vi "vdP_measurement.vi"() -> ()   [LabVIEW 2026]
uses:
  <vilib>/regexp/Match Regular Expression.xnode
panel:
  out "rho (Ohm * m)":dbl
  out "Rs (Ohm/sq)":dbl
  in  "VISA resource name":refnum<visa-resource-name>="TCPIP0::192.168.0.4::1225::SOCKET"
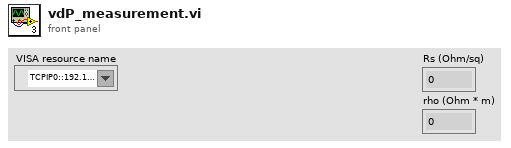
[diagram p1: front panel]
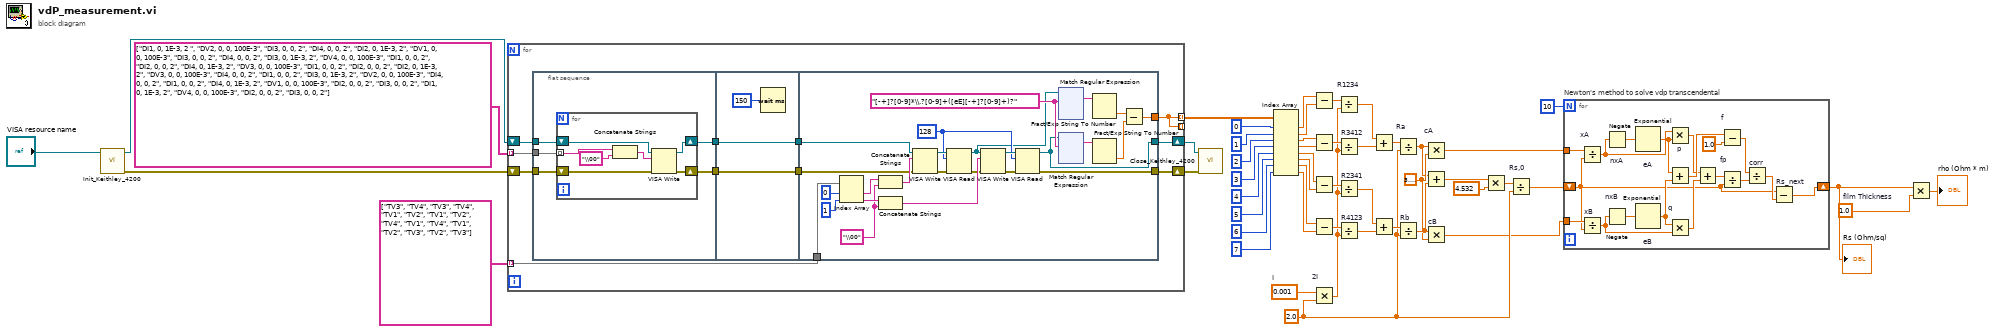
[diagram p0: block diagram]
diagram:
  w9 = 3.141592653589793
  w2 = 1.0  # film Thickness
  w34 = 0.001  # I
  w11 = 2.0 ("y")
  n1 = call "Init_Keithley_4200.vi"("VISA resource name"="VISA resource name") -> ("error out"=w46:errorcluster, "VISA resource name out"=w47:refnum<visa-resource-name>)  [unwired: 9 in]
  n2 = for {
    tunnel: string[][] [["DI1, 0, 1E-3, 2 ", "DV2, 0, 0, 100E-3", "DI3, 0, 0, 2", "DI4, 0, 0, 2"], ["DI2, 0, 1E-3, 2", "DV1, 0, 0, 100E-3", "DI3, 0, 0, 2", "DI4, 0, 0, 2"], ["DI3, 0, 1E-3, 2", "DV4, 0, 0, 100E-3", "DI1, 0, 0, 2", "DI2, 0, 0, 2"], ["DI4, 0, 1E-3, 2", "DV3, 0, 0, 100E-3", "DI1, 0, 0, 2", "DI2, 0, 0, 2"], ["DI2, 0, 1E-3, 2", "DV3, 0, 0, 100E-3", "DI4, 0, 0, 2", "DI1, 0, 0, 2"], ["DI3, 0, 1E-3, 2", "DV2, 0, 0, 100E-3", "DI4, 0, 0, 2", "DI1, 0, 0, 2"], ["DI4, 0, 1E-3, 2", "DV1, 0, 0, 100E-3", "DI2, 0, 0, 2", "DI3, 0, 0, 2"], ["DI1, 0, 1E-3, 2", "DV4, 0, 0, 100E-3", "DI2, 0, 0, 2", "DI3, 0, 0, 2"]] -> [w58] mode=indexing
    tunnel: string[][] [["TV3", "TV4"], ["TV3", "TV4"], ["TV1", "TV2"], ["TV1", "TV2"], ["TV4", "TV1"], ["TV4", "TV1"], ["TV2", "TV3"], ["TV2", "TV3"]] -> [w59] mode=indexing
    shift-right: [w52] -> w45
    shift-left: w47 -> [w61]
    shift-right: [w53] -> w44
    shift-left: w46 -> [w60]
    tunnel: [w51] -> _ mode=indexing
    tunnel: [w51] -> w43 mode=indexing
    n3 = flat-sequence {
      tunnel: w61 -> [w65]
      tunnel: w60 -> [w64]
      tunnel: w58 -> [w66]
      tunnel: [w63] -> w57
      tunnel: [w62] -> w56
      tunnel: w57 -> [w75]
      tunnel: w56 -> [w74]
      tunnel: [w75] -> w55
      tunnel: [w74] -> w54
      tunnel: w59 -> [w101]
      tunnel: w55 -> [w91]
      tunnel: w54 -> [w90]
      tunnel: [w81] -> w51
      tunnel: [w78] -> w53
      tunnel: [w77] -> w52
      frame #0 {
        n4 = for {
          tunnel: w66 -> [w73] mode=indexing
          shift-right: [w68] -> w63
          shift-left: w65 -> [w71]
          shift-right: [w67] -> w62
          shift-left: w64 -> [w69]
          n5 = Concatenate Strings(w73, "\\00") -> (w70:string)
          n6 = VISA Write(VISA resource name=w71, write buffer=w70, error in (no error)=w69) -> (VISA resource name out=w68:refnum<visa-resource-name>, error out=w67:errorcluster)  [unwired: 1 out]
        }
      }
      frame #1 {
        n7 = Wait (ms)(milliseconds to wait=u32 150) -> ()  [unwired: 1 out]
      }
      frame #2 {
        w86 = "[-+]?[0-9]*\\.?[0-9]+([eE][-+]?[0-9]+)?" ("regular expression")
        w87 = u32 128 ("byte count")
        w93 = "\\00"
        n8 = Index Array(array=w101, index #1=0 ("index"), index #2=1 ("index")) -> (element #1=w96:string, element #2=w94:string)
        n9 = Concatenate Strings(w96, w93) -> (w95:string)
        n10 = Concatenate Strings(w94, w93) -> (w92:string)
        n11 = VISA Write(VISA resource name=w91, write buffer=w95, error in (no error)=w90) -> (VISA resource name out=w97:refnum<visa-resource-name>, error out=w98:errorcluster)  [unwired: 1 out]
        n12 = VISA Read(VISA resource name=w97, byte count=w87, error in (no error)=w98) -> (VISA resource name out=w80:refnum<visa-resource-name>, error out=w79:errorcluster)  [unwired: 2 out]
        n13 = VISA Write(VISA resource name=w80, write buffer=w92, error in (no error)=w79) -> (VISA resource name out=w89:refnum<visa-resource-name>, error out=w88:errorcluster)  [unwired: 1 out]
        n14 = VISA Read(VISA resource name=w89, byte count=w87, error in (no error)=w88) -> (VISA resource name out=w77:refnum<visa-resource-name>, error out=w78:errorcluster)  [unwired: 2 out]
        n15 = xnode "Match Regular Expression"("input string"=w80, "regular expression"=w86) -> ("whole match"=w85:string)  [unwired: 4 in, 4 out]
        n16 = xnode "Match Regular Expression"("input string"=w77, "regular expression"=w86) -> ("whole match"=w84:string)  [unwired: 4 in, 4 out]
        n17 = Fract/Exp String To Number(string=w85) -> (number=w83:dbl)  [unwired: 3 in, 1 out]
        n18 = Fract/Exp String To Number(string=w84) -> (number=w82:dbl)  [unwired: 3 in, 1 out]
        n19 = Subtract(x=w83, y=w82) -> (x-y=w81:dbl)
      }
    }
  }
  n20 = call "Close_Keithley_4200.vi"("error in (no error)"=w44, "VISA resource name"=w45) -> ()  [unwired: 9 in, 1 out]
  n21 = Index Array(array=w43, index #1=0 ("index"), index #2=1 ("index"), index #3=2 ("index"), index #4=3 ("index"), index #5=4 ("index"), index #6=5 ("index"), index #7=6 ("index"), index #8=7 ("index")) -> (element #1=w33:dbl, element #2=w32:dbl, element #3=w31:dbl, element #4=w30:dbl, element #5=w29:dbl, element #6=w28:dbl, element #7=w27:dbl, element #8=w26:dbl)
  n22 = Subtract(x=w33, y=w32) -> (x-y=w25:dbl)
  n23 = Subtract(x=w31, y=w30) -> (x-y=w24:dbl)
  n24 = Subtract(x=w29, y=w28) -> (x-y=w23:dbl)
  n25 = Subtract(x=w27, y=w26) -> (x-y=w22:dbl)
  n26 = Multiply "2I"(x=w34, y=w11) -> (x*y=w21:dbl)
  n27 = Divide "R1234"(x=w25, y=w21) -> (x/y=w20:dbl)
  n28 = Divide "R3412"(x=w24, y=w21) -> (x/y=w19:dbl)
  n29 = Divide "R2341"(x=w23, y=w21) -> (x/y=w18:dbl)
  n30 = Divide "R4123"(x=w22, y=w21) -> (x/y=w17:dbl)
  n31 = Add(x=w20, y=w19) -> (x+y=w16:dbl)
  n32 = Add(x=w18, y=w17) -> (x+y=w15:dbl)
  n33 = Divide "Ra"(x=w16, y=w11) -> (x/y=w8:dbl)
  n34 = Divide "Rb"(x=w15, y=w11) -> (x/y=w10:dbl)
  n35 = Multiply "cA"(x=w8, y=w9) -> (x*y=w5:dbl)
  n36 = Add(x=w8, y=w10) -> (x+y=w14:dbl)
  n37 = Multiply "cB"(x=w10, y=w9) -> (x*y=w4:dbl)
  n38 = Multiply(x=w14, y=4.532) -> (x*y=w13:dbl)
  n39 = Divide "Rs,0"(x=w13, y=w11) -> (x/y=w6:dbl)
  n40 = for "Newton's method to solve vdp transcendental" {
    N: 10 -> [_]
    shift-right: [w336] -> w3
    shift-left: w6 -> [w337]
    tunnel: w5 -> [w353]
    tunnel: w4 -> [w352]
    n41 = Divide "xA"(x=w353, y=w337) -> (x/y=w347:dbl)
    n42 = Divide "xB"(x=w352, y=w337) -> (x/y=w345:dbl)
    n43 = Negate "nxA"(x=w347) -> (-x=w351:dbl)
    n44 = Negate "nxB"(x=w345) -> (-x=w350:dbl)
    n45 = Exponential "eA"(1:w351) -> (0:w346:dbl)
    n46 = Exponential "eB"(1:w350) -> (0:w344:dbl)
    n47 = Multiply "p"(x=w347, y=w346) -> (x*y=w343:dbl)
    n48 = Add(x=w346, y=w344) -> (x+y=w349:dbl)
    n49 = Multiply "q"(x=w344, y=w345) -> (x*y=w342:dbl)
    n50 = Add(x=w343, y=w342) -> (x+y=w341:dbl)
    n51 = Subtract "f"(x=w349, y=1.0) -> (x-y=w340:dbl)
    n52 = Divide "fp"(x=w341, y=w337) -> (x/y=w339:dbl)
    n53 = Divide "corr"(x=w340, y=w339) -> (x/y=w338:dbl)
    n54 = Subtract "Rs_next"(x=w337, y=w338) -> (x-y=w336:dbl)
  }
  "Rs (Ohm/sq)" <- w3
  n55 = Multiply(x=w3, y=w2) -> (x*y=→"rho (Ohm * m)":dbl)
